vi "Get Fullpath.vi"(8 "error in (no error)":errorcluster, 11 "TreeNode in":refnum<class "TreeNode.lvclass">) -> (0 "error out":errorcluster, 2 "Fullpath":string, 3 "TreeNode out":refnum<class "TreeNode.lvclass">)   [LabVIEW 2015, in "MDSplus.lvlib" / "TreeNode.lvclass"]
uses:
  <vilib>/MDSplus/Classes/Data_Class/TreeNode_Class/TreeNode.lvclass
  MDSobjectsLVShr.dll
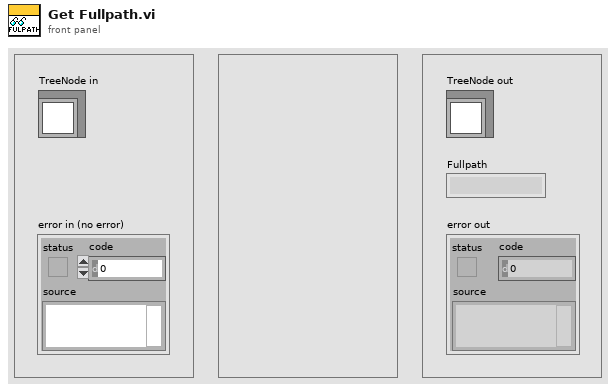
[diagram p1: front panel]
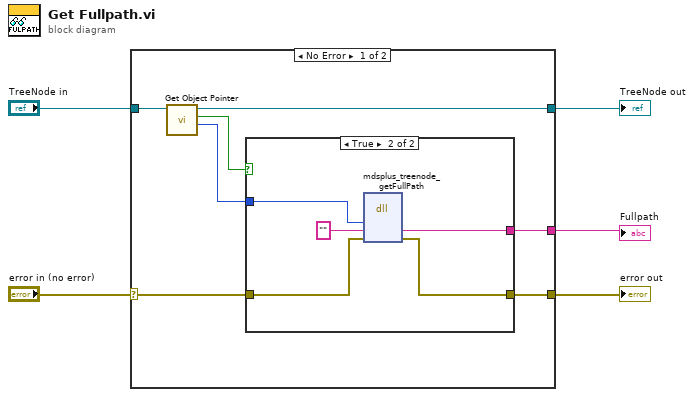
[diagram p0: block diagram]
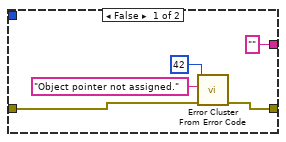
[diagram p2: hidden frame]
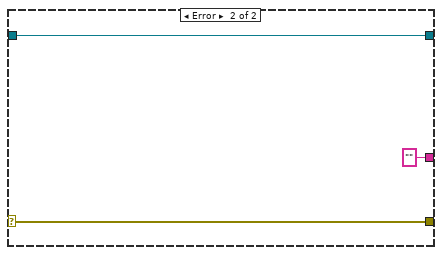
[diagram p3: hidden frame]
diagram:
  n1 = case shown="No Error" "error in (no error)" {
    selector: "error in (no error)" -> [w11 w25]
    tunnel: [w12 w25] -> w4
    tunnel: [w10 "" ("lvStrHdlOut")] -> w3
    tunnel: "TreeNode in" -> [w9 w24]
    tunnel: [w8 w24] -> w1
    frame No Error {
      n2 = call-dynamic "Get Object Pointer.vi"("Data in"=w9) -> ("Object Pointer"=w6:i64, "Assigned object pointer?"=w7:bool, "Data out"=w8:refnum<class "TreeNode.lvclass">)  [unwired: 8 in]
      n3 = case shown="True" w7 {
        tunnel: ["" ("sizeOut") w22] -> w10
        tunnel: w6 -> [_ w20]
        tunnel: w11 -> [w14 w19]
        tunnel: [w13 w18] -> w12
        frame False {
          n4 = call <vilib>:"Error Cluster From Error Code.vi"("error in (no error)"=w14, "error message (\"\")"="Object pointer not assigned." ("error message (\"\")"), "error code (0)"=42) -> ("error out"=w13:errorcluster)  [unwired: 6 in]
        }
        frame True {
          n5 = dll-call lib="MDSobjectsLVShr.dll" fn="mdsplus_treenode_getFullPath"("lvTreeNodePtr"=w20, "lvStrHdlOut"="" ("size"), "error"=w19) -> ("lvStrHdlOut"=w22:string, "error"=w18:errorcluster)  [unwired: 5 in, 2 out]
        }
      }
    }
    frame Error {
    }
  }
  "error out" <- w4
  "TreeNode out" <- w1
  "Fullpath" <- w3
